vi "ZLIB Open Unzip__ogtk.vi"   [LabVIEW 2011]
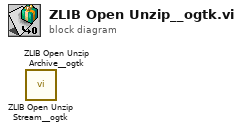
[diagram p0: block diagram]
diagram:
  n1 = call "ZLIB Open Unzip Stream__ogtk.vi"() -> ()  [unwired: 6 in, 2 out]
  n2 = call "ZLIB Open Unzip Archive__ogtk.vi"() -> ()  [unwired: 6 in, 2 out]
